vi "Dispose.vi"(8 "error in (no error)":errorcluster, 11 "WebView2 Control in":refnum<class "WebView2 QControl.lvclass">) -> (0 "error out":errorcluster)   [LabVIEW 2020, in "WebView2 QControl.lvlib" / "WebView2 QControl.lvclass"]
uses:
  WebView2 QControl.lvclass
  WebView2 QControl.lvclass/WebView2 QControl.ctl
  Webview2 Lib/WebView2 Control Object/WebView2 Control.lvclass
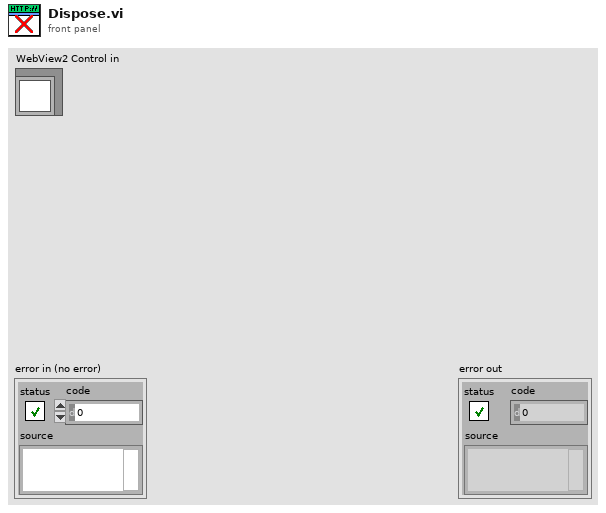
[diagram p1: front panel]
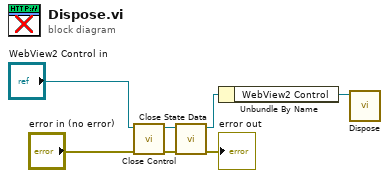
[diagram p0: block diagram]
diagram:
  n1 = call-dynamic "Close Control.vi"("error in (no error)"="error in (no error)", "Control in"="WebView2 Control in") -> ("error out"=w4:errorcluster, "Control out"=w2:refnum<class "WebView2 QControl.lvclass">)  [unwired: 8 in]
  n2 = call-dynamic "Close State Data.vi"("error in (no error)"=w4, "Control in"=w2) -> ("error out"=→"error out":errorcluster, "Control out"=w1:refnum<class "WebView2 QControl.lvclass">)  [unwired: 8 in]
  n3 = Unbundle By Name(w1) -> ("WebView2 Control"=w7:refnum<class "WebView2 Control.lvclass">)
  n4 = call "Dispose.vi"("WebView2 Control in"=w7) -> ()  [unwired: 10 in, 1 out]
